vi "Serrure_V2_2fichier.vi"() -> ()   [LabVIEW 2018]
panel:
  in  "Compteur":i8 min=0 max=5
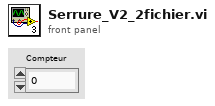
[diagram p1: front panel]
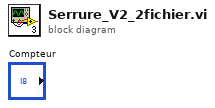
[diagram p0: block diagram]
diagram:
